vi "Caculate_intension.vi"(0 "w2":i32, 1 "w1":i32, 2 "file path":path, 3 "h2":i32, 4 "h1":i32, 5 "Boolean":bool, 6 "img_data":dbl[][](array[numeric])) -> ()   [LabVIEW 2016]
panel:
  out "Intension":dbl
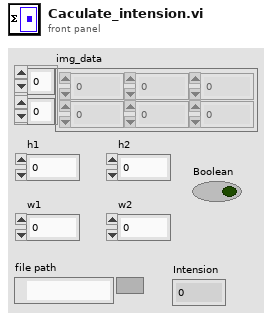
[diagram p1: front panel]
types:
  T1 = enum16{"open", "replace", "create", "open or create", "replace or create", "replace or create with confirmation"}
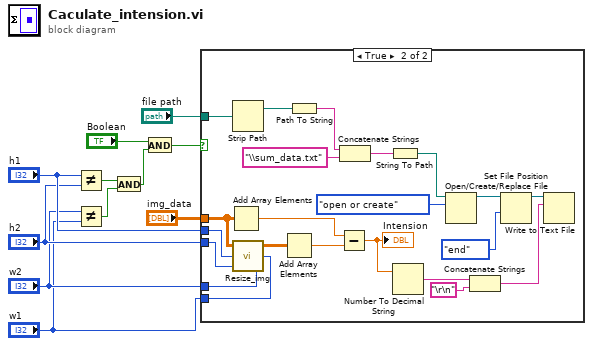
[diagram p0: block diagram]
diagram:
  n1 = Not Equal?(x="h1", y="h2") -> (x != y?=w2:bool)
  n2 = Not Equal?(x="w2", y="w1") -> (x != y?=w3:bool)
  n3 = And(x=w2, y=w3) -> (x .and. y?=w1:bool)
  n4 = And(x="Boolean", y=w1) -> (x .and. y?=w8:bool)
  n5 = case shown="True" w8 {
    tunnel: "img_data" -> [_ w33]
    tunnel: "h1" -> [_ w29]
    tunnel: "h2" -> [_ w28]
    tunnel: "w1" -> [_ w27]
    tunnel: "w2" -> [_ w26]
    tunnel: "file path" -> [_ w15]
    frame False {
    }
    frame True {
      n6 = Add Array Elements(numeric array=w33) -> (sum=w31:dbl)
      n7 = Strip Path(path=w15) -> (stripped path=w16:path)  [unwired: 1 out]
      n8 = call "Resize_img.vi"("w2"=w26, "w1"=w27, "h2"=w28, "h1"=w29, "img_in"=w33) -> ("img_out"=w32:dbl[][])
      n9 = Add Array Elements(numeric array=w32) -> (sum=w30:dbl)
      n10 = Path To String(path=w16) -> (string=w19:string)
      n11 = Subtract(x=w31, y=w30) -> (x-y=w25:dbl)
      "Intension" <- w25
      n12 = Concatenate Strings(w19, "\\sum_data.txt" ("regular expression (\"\")")) -> (w20:string)
      n13 = String To Path(string=w20) -> (path=w17:path)
      n14 = Number To Decimal String(number=w25) -> (decimal integer string=w13:string)  [unwired: 1 in]
      n15 = Open/Create/Replace File(file path (use dialog)=w17, operation (0:open)=T1."open or create") -> (refnum out=w22:refnum<file>)  [unwired: 4 in, 2 out]
      n16 = Concatenate Strings(w13, "\r\n") -> (w12:string)
      n17 = Set File Position(refnum=w22, from (0:start)=enum16{"start", "end", "current"}."end") -> (refnum out=w24:refnum<file>)  [unwired: 2 in, 1 out]
      n18 = Write to Text File(file (use dialog)=w24, text=w12) -> ()  [unwired: 2 in, 3 out]
    }
  }
